vi "OpenAppIfInputDefault.vi"(8 "error in (no error)":errorcluster, 11 "Application":refnum<vi>) -> (0 "error out":errorcluster, 2 "New app opened?":bool, 3 "valid application reference":refnum<vi>)   [LabVIEW 2019, in "BlueUtilityScripts.lvlib"]
uses:
  BlueUtilityScripts.lvlib
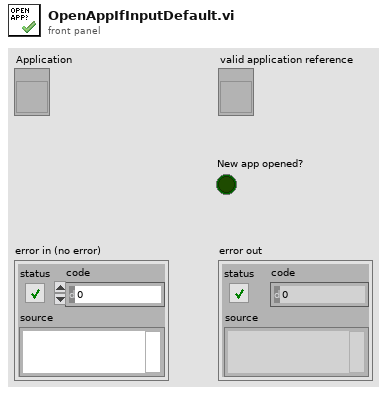
[diagram p1: front panel]
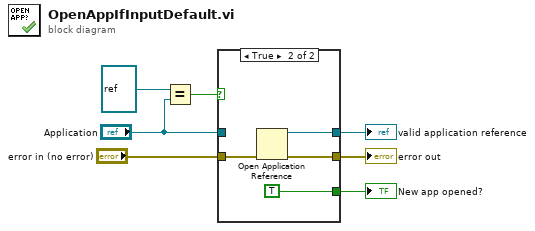
[diagram p0: block diagram]
diagram:
  n1 = Equal?(x=refnum<vi> refnum ("Application"), y="Application") -> (x = y?=w6:bool)
  n2 = case shown="True" w6 {
    tunnel: "Application" -> [w9 _]
    tunnel: [w9 w13] -> w2
    tunnel: "error in (no error)" -> [w8 w12]
    tunnel: [w8 w11] -> w3
    tunnel: [_ TRUE] -> w1
    frame False {
    }
    frame True {
      n3 = Open Application Reference(8:w12) -> (0:w11:errorcluster, 3:w13:refnum<vi>)  [unwired: 3 in]
    }
  }
  "error out" <- w3
  "valid application reference" <- w2
  "New app opened?" <- w1
